vi "set all outputs.vi"(6 "wait for reply (T)":bool=TRUE, 7 "Output On/Off":bool, 8 "error in":errorcluster, 9 "Current":dbl, 10 "Voltage":dbl, 11 "Module ID":i32=-1) -> (0 "error out":errorcluster, 1 "timed out?":bool)   [LabVIEW 2025, in "Power Supply.lvlib"]
doc: "_____\nCreated using DQMH Framework: Event Scripter 7.1.2.1547."
uses:
  Power Supply.lvlib
  set all outputs Argument--cluster.ctl
  set all outputs (Reply Payload)--cluster.ctl
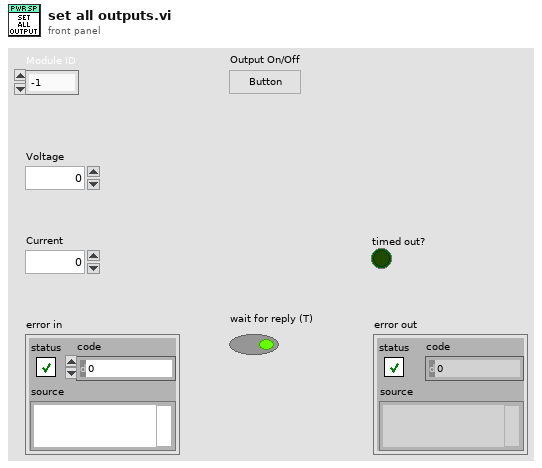
[diagram p1: front panel]
types:
  T1 = typedef "Power Supply.lvlib/set all outputs Argument--cluster.ctl" = cluster{"Module ID":i32, "Voltage":dbl, "Current":dbl, "Output On/Off":bool, "Wait Notifier":refnum<notifier>, "wait for reply":bool}
  T2 = typedef "Power Supply.lvlib/Request Events--cluster.ctl" = cluster{"Stop Module":refnum<user-event>, "Show Panel":refnum<user-event>, "Hide Panel":refnum<user-event>, "Show Diagram":refnum<user-event>, "Get Module Execution Status":refnum<user-event>, "select child":refnum<user-event>, "read config":refnum<user-event>, "init device":refnum<user-event>, "close":refnum<user-event>, "output":refnum<user-event>, "set voltage":refnum<user-event>, "set current":refnum<user-event>, "read current":refnum<user-event>, "read voltage":refnum<user-event>, "read state":refnum<user-event>, "set all outputs":refnum<user-event>}
  T3 = typedef "Power Supply.lvlib/set all outputs (Reply Payload)--cluster.ctl" = cluster{"Module ID":i32, "error":errorcluster}
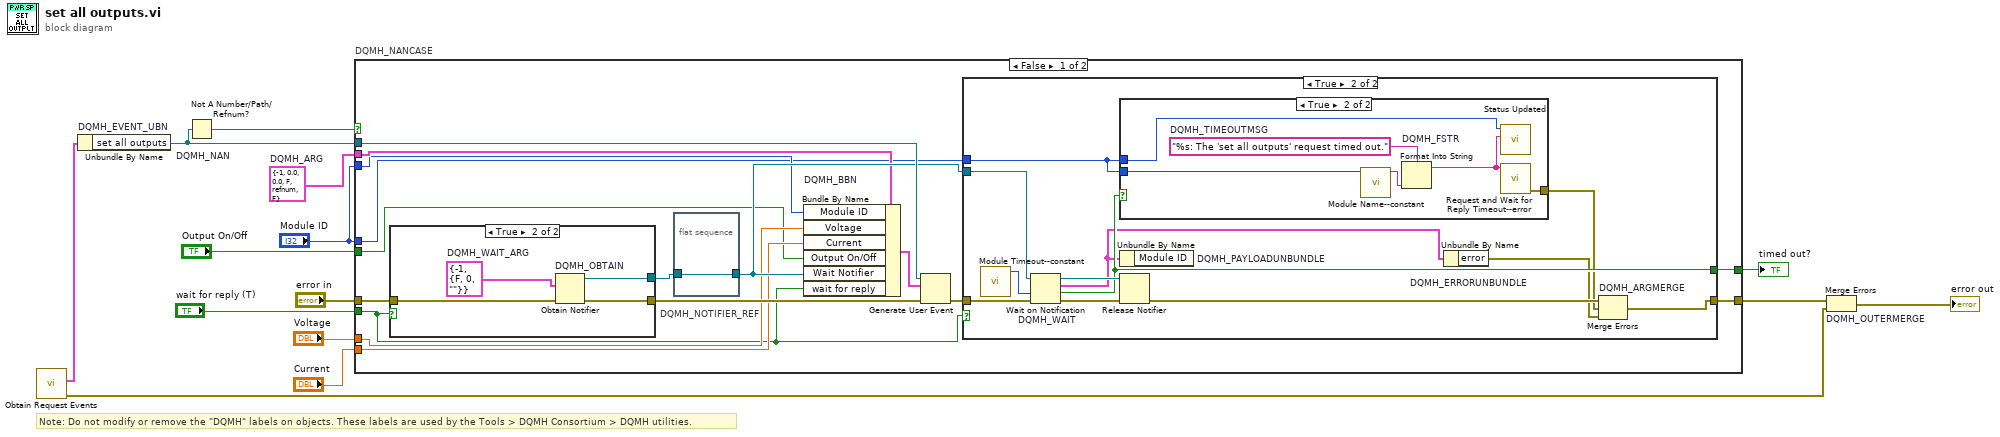
[diagram p0: block diagram]
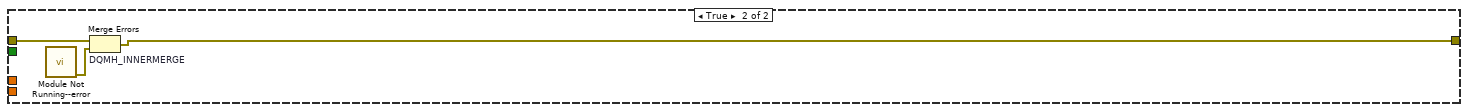
[diagram p5: hidden frame]
diagram:
  w8 = T1 {"Module ID"=-1, "Voltage"=0.0, "Current"=0.0, "Output On/Off"=FALSE, "Wait Notifier"=refnum, "wait for reply"=FALSE}  # DQMH_ARG
  # "Note: Do not modify or remove the \"DQMH\" labels on objects. These labels are used by the Tools > DQMH Consortium > DQMH utilities."
  n1 = call "Obtain Request Events.vi"() -> ("error out"=w2:errorcluster, "Power Supply Request Events"=w1:T2)  [unwired: 10 in]
  n2 = Unbundle By Name "DQMH_EVENT_UBN"(w1) -> ("set all outputs"=w12:refnum<user-event>)
  n3 = Not A Number/Path/Refnum? "DQMH_NAN"(number/path/refnum=w12) -> (NaN/Path/Refnum?=w11:bool)
  n4 = case "DQMH_NANCASE" shown="False" w11 {
    tunnel: "error in" -> [w30 w58]
    tunnel: w12 -> [w28 _]
    tunnel: [w25 w57] -> w9
    tunnel: [w26 _] -> w10
    tunnel: w8 -> [w21 _]
    tunnel: "Module ID" -> [w20 _]
    tunnel: "Voltage" -> [w19 _]
    tunnel: "Current" -> [w18 _]
    tunnel: "Output On/Off" -> [w17 _]
    tunnel: "Module ID" -> [w16 _]
    tunnel: "wait for reply (T)" -> [w15 _]
    frame False {
      n5 = case shown="True" w15 {
        tunnel: w30 -> [w51 w55]
        tunnel: [w51 w54] -> w27
        tunnel: [_ w52] -> w23
        frame False {
        }
        frame True {
          w53 = T3 {"Module ID"=-1, "error"={"status"=FALSE, "code"=0, "source"=""}}  # DQMH_WAIT_ARG
          n6 = Obtain Notifier "DQMH_OBTAIN"(notification data type=w53, error in (no error)=w55) -> (notifier out=w52:refnum<notifier>, error out=w54:errorcluster)  [unwired: 2 in, 1 out]
        }
      }
      n7 = flat-sequence "DQMH_NOTIFIER_REF" {
        tunnel: w23 -> [w31]
        tunnel: [w31] -> w22
        frame #0 {
        }
      }
      n8 = Bundle By Name "DQMH_BBN"(cluster=w21, "Module ID"=w20, "Voltage"=w19, "Current"=w18, "Output On/Off"=w17, "Wait Notifier"=w22, "wait for reply"=w15) -> (w24:T1)
      n9 = Generate User Event(user event=w28, event data cluster=w24, error in=w27) -> (error out=w29:errorcluster)  [unwired: 1 in, 1 out]
      n10 = case shown="True" w15 {
        tunnel: w29 -> [w32 w44]
        tunnel: w22 -> [_ w43]
        tunnel: [_ w41] -> w26
        tunnel: [w32 w40] -> w25
        tunnel: w16 -> [_ w33]
        frame False {
        }
        frame True {
          n11 = call "Module Timeout--constant.vi"() -> ("Module Timeout"=w34:i32)  [unwired: 11 in]
          n12 = Wait on Notification "DQMH_WAIT"(notifier=w43, timeout in ms (-1)=w34, error in (no error)=w44) -> (notifier out=w42:refnum<notifier>, notification=w35:T3, timed out?=w41:bool, error out=w39:errorcluster)  [unwired: 1 in]
          n13 = case shown="True" w41 {
            tunnel: [_ w48] -> w36
            tunnel: w33 -> [_ w46]
            tunnel: w33 -> [_ w45]
            frame False {
            }
            frame True {
              w50 = "%s: The 'set all outputs' request timed out."  # DQMH_TIMEOUTMSG
              n14 = call "Module Name--constant.vi"("Module ID"=w45) -> ("Module Name"=w47:string)  [unwired: 10 in]
              n15 = Format Into String "DQMH_FSTR"(format string=w50, w47) -> (resulting string=w49:string)  [unwired: 2 in, 1 out]
              n16 = call "Status Updated.vi"("Status"=w49, "Module ID"=w46) -> ()  [unwired: 9 in, 1 out]
              n17 = call "Request and Wait for Reply Timeout--error.vi"("Error Message"=w49) -> ("error out"=w48:errorcluster)  [unwired: 10 in]
            }
          }
          n18 = Unbundle By Name "DQMH_PAYLOADUNBUNDLE"(w35) -> ()  [unwired: 1 out]
          n19 = Release Notifier(notifier=w42, error in (no error)=w39) -> (error out=w38:errorcluster)  [unwired: 1 in, 2 out]
          n20 = Unbundle By Name "DQMH_ERRORUNBUNDLE"(w35) -> ("error"=w37:errorcluster)
          n21 = Merge Errors "DQMH_ARGMERGE"(w38, w36, w37) -> (w40:errorcluster)
        }
      }
    }
    frame True {
      n22 = call "Module Not Running--error.vi"() -> ("error out"=w56:errorcluster)  [unwired: 11 in]
      n23 = Merge Errors "DQMH_INNERMERGE"(w58, w56) -> (w57:errorcluster)
    }
  }
  "timed out?" <- w10
  n24 = Merge Errors "DQMH_OUTERMERGE"(w9, w2) -> (→"error out":errorcluster)
